vi "SelectPoint.vi"(10 "PointName":string="PT", 11 "RobotPointsTableIn":string[][](table)) -> (1 "Count":i32, 2 "RobotPointsOut":string[][](table), 3 "RobotPointsTableOut":string[][](table))   [LabVIEW 2014]
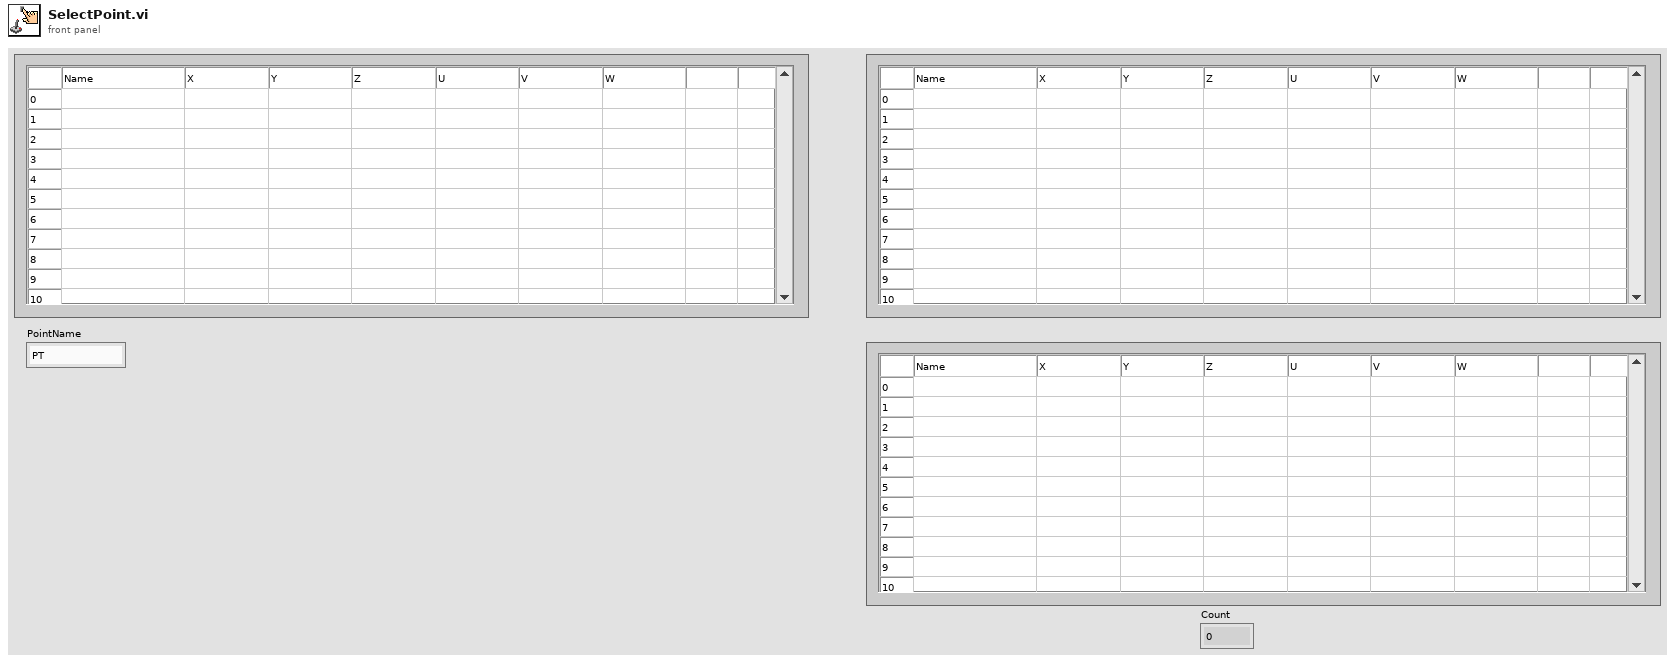
[diagram p1: front panel]
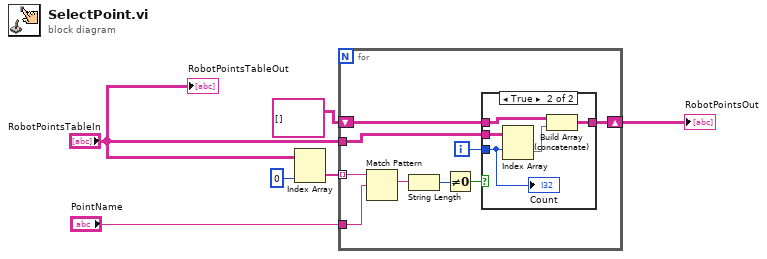
[diagram p0: block diagram]
diagram:
  n1 = Index Array(array="RobotPointsTableIn", index (col)=0 ("disabled index (col)")) -> (element=w5:string[])  [unwired: 1 in]
  n2 = for {
    tunnel: w5 -> [w15] mode=indexing
    tunnel: "PointName" -> [w14]
    tunnel: "RobotPointsTableIn" -> [w9]
    shift-right: [w7] -> w1
    shift-left: string[][] [] -> [w8]
    i -> [w13]
    n3 = Match Pattern(string=w15, regular expression=w14) -> (match substring=w11:string)  [unwired: 1 in, 3 out]
    n4 = String Length(string=w11) -> (length=w10:i32)
    n5 = Not Equal To 0?(x=w10) -> (x != 0?=w12:bool)
    n6 = case shown="True" w12 {
      tunnel: w13 -> [_ w20]
      tunnel: w9 -> [_ w21]
      tunnel: w8 -> [w16 w19]
      tunnel: [w16 w17] -> w7
      frame False {
      }
      frame True {
        n7 = Index Array(array=w21, index (row)=w20) -> (element=w18:string[])  [unwired: 1 in]
        n8 = Build Array (concatenate)(w19, w18) -> (w17:string[][])
        "Count" <- w20
      }
    }
  }
  "RobotPointsOut" <- w1
  "RobotPointsTableOut" <- "RobotPointsTableIn"
